vi "phasePlotWrap.vi"(6 "Sampling info":cluster{"Fs":dbl, "#s":dbl}={"Fs"=10000.0, "#s"=1000.0} {"Fs" format="%.2p"}, 8 "Phase Unit":u16(ring) items=["Degree", "Radian"], 9 "Input phase":dbl, 10 "Input frequency":dbl=50.0, 11 "Nominal Frequency":dbl=50.0) -> (3 "Phase waveform":waveform(dbl)(graph))   [LabVIEW 2025]
uses:
  <vilib>/measure/NI_MAPro.lvlib
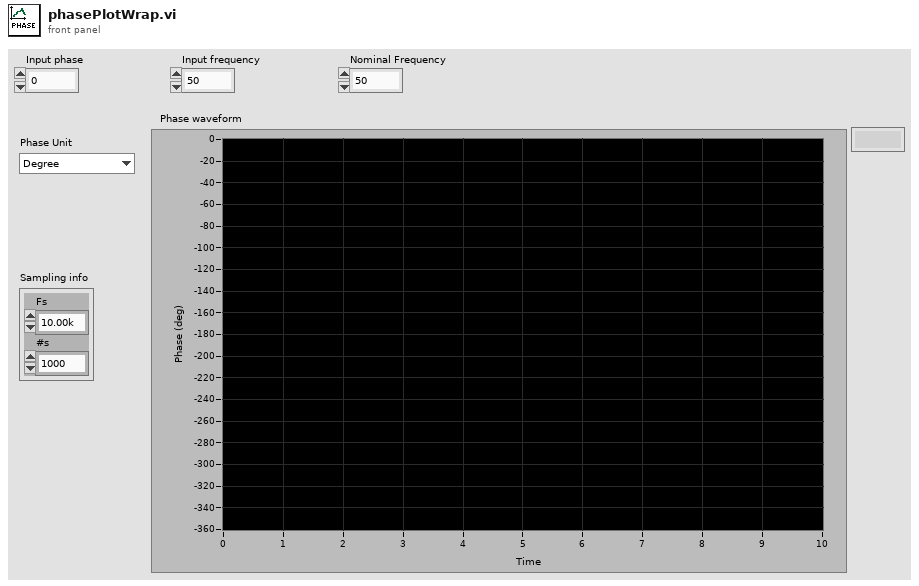
[diagram p1: front panel]
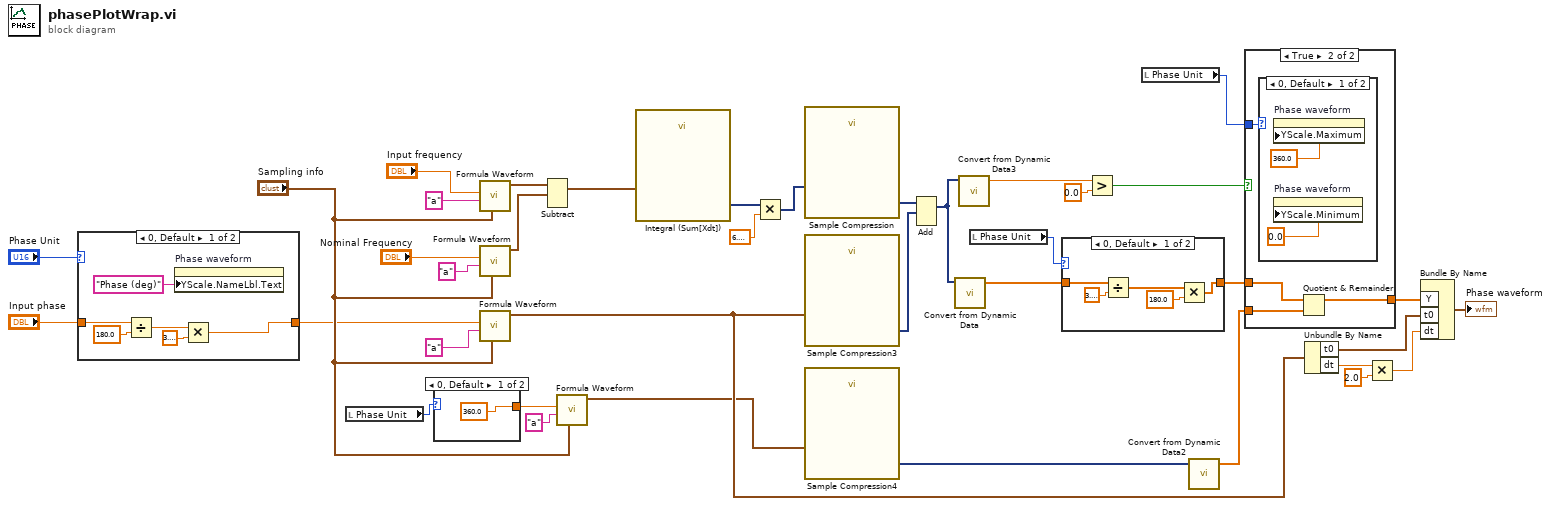
[diagram p0: block diagram]
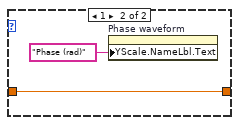
[diagram p2: hidden frame]
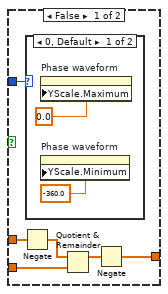
[diagram p3: hidden frame]
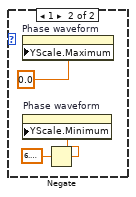
[diagram p4: hidden frame]
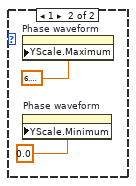
[diagram p5: hidden frame]
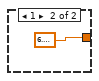
[diagram p6: hidden frame]
diagram:
  n1 = case shown="0, Default" "Phase Unit" {
    tunnel: "Input phase" -> [w42 w45]
    tunnel: [w39 w45] -> w1
    frame 0, Default {
      n2 = Divide(x=w42, y=180.0) -> (x/y=w41:dbl)
      n3 = property on="Phase waveform" class="WFChart (strict)"("YScale.NameLbl.Text"="Phase (deg)" ("Y Scale.Name Label.Text")) -> ()  [unwired: 2 in, 2 out]
      n4 = Multiply(x=w41, y=3.141592653589793) -> (x*y=w39:dbl)
    }
    frame 1 {
      n5 = property on="Phase waveform" class="WFChart (strict)"("YScale.NameLbl.Text"="Phase (rad)" ("Y Scale.Name Label.Text")) -> ()  [unwired: 2 in, 2 out]
    }
  }
  n6 = local read "Phase Unit"() -> (w21:u16)
  n7 = case shown="0, Default" w21 {
    tunnel: [360.0 6.283185307179586] -> w22
    frame 0, Default {
    }
    frame 1 {
    }
  }
  n8 = call <vilib>:"Formula Waveform.vi"("sampling info"="Sampling info", "formula"="a", "amplitude"="Input frequency") -> ("signal out"=w14:waveform(dbl))  [unwired: 7 in, 1 out]
  n9 = call <vilib>:"Formula Waveform.vi"("sampling info"="Sampling info", "formula"="a", "amplitude"="Nominal Frequency") -> ("signal out"=w15:waveform(dbl))  [unwired: 7 in, 1 out]
  n10 = call <vilib>:"Formula Waveform.vi"("sampling info"="Sampling info", "formula"="a", "amplitude"=w1) -> ("signal out"=w31:waveform(dbl))  [unwired: 7 in, 1 out]
  n11 = Subtract(1:w15, 2:w14) -> (0:w16:waveform(dbl))  [unwired: 1 in, 1 out]
  n12 = call <vilib>:"Formula Waveform.vi"("sampling info"="Sampling info", "formula"="a", "amplitude"=w22) -> ("signal out"=w20:waveform(dbl))  [unwired: 7 in, 1 out]
  n13 = call "Integral (Sum[Xdt])"("Signals"=w16) -> ("Result"=w12:dynamicdata)  [unwired: 5 in, 1 out]
  n14 = Multiply(x=w12, y=6.283185307179586) -> (x*y=w10:dynamicdata)
  n15 = call "Sample Compression"("Signals"=w10) -> ("Maximum"=w11:dynamicdata)  [unwired: 8 in, 2 out]
  n16 = call "Sample Compression3"("Signals"=w31) -> ("Maximum"=w27:dynamicdata)  [unwired: 8 in, 2 out]
  n17 = call "Sample Compression4"("Signals"=w20) -> ("Maximum"=w30:dynamicdata)  [unwired: 8 in, 2 out]
  n18 = Add(1:w27, 2:w11) -> (0:w36:dynamicdata)  [unwired: 1 in, 1 out]
  n19 = call "Convert from Dynamic Data"("Dynamic Data Type"=w36) -> ("Array"=w24:dbl[])  [unwired: 3 in]
  n20 = call "Convert from Dynamic Data3"("Dynamic Data Type"=w36) -> ("Scalar"=w37:dbl)  [unwired: 3 in]
  n21 = local read "Phase Unit"() -> (w9:u16)
  n22 = case shown="0, Default" w9 {
    tunnel: w24 -> [w53 w54]
    tunnel: [w50 w54] -> w23
    frame 0, Default {
      n23 = Divide(x=w53, y=3.141592653589793) -> (x/y=w52:dbl[])
      n24 = Multiply(x=w52, y=180.0) -> (x*y=w50:dbl[])
    }
    frame 1 {
    }
  }
  n25 = Greater?(x=w37, y=0.0) -> (0:w26:bool)
  n26 = local read "Phase Unit"() -> (w38:u16)
  n27 = call "Convert from Dynamic Data2"("Dynamic Data Type"=w30) -> ("Array"=w25:dbl[])  [unwired: 3 in]
  n28 = case shown="True" w26 {
    tunnel: w23 -> [w59 w69]
    tunnel: w25 -> [w58 w68]
    tunnel: [w57 w67] -> w28
    tunnel: w38 -> [w55 w66]
    frame False {
      n29 = Negate(x=w59) -> (-x=w60:dbl[])
      n30 = case shown="0, Default" w55 {
        frame 0, Default {
          n31 = property on="Phase waveform" class="WFChart (strict)"("YScale.Maximum"=0.0 ("Y Scale.Range:Maximum")) -> ()  [unwired: 2 in, 2 out]
          n32 = property on="Phase waveform" class="WFChart (strict)"("YScale.Minimum"=-360.0 ("Y Scale.Range:Minimum")) -> ()  [unwired: 2 in, 2 out]
        }
        frame 1 {
          n33 = property on="Phase waveform" class="WFChart (strict)"("YScale.Maximum"=0.0 ("Y Scale.Range:Minimum")) -> ()  [unwired: 2 in, 2 out]
          n34 = Negate(x=6.283185307179586) -> (-x=w63:dbl)
          n35 = property on="Phase waveform" class="WFChart (strict)"("YScale.Minimum"=w63) -> ()  [unwired: 2 in, 2 out]
        }
      }
      n36 = Quotient & Remainder(x=w60, y=w58) -> (x-y*floor(x/y)=w56:dbl[])  [unwired: 1 out]
      n37 = Negate(x=w56) -> (-x=w57:dbl[])
    }
    frame True {
      n38 = case shown="0, Default" w66 {
        frame 0, Default {
          n39 = property on="Phase waveform" class="WFChart (strict)"("YScale.Maximum"=360.0 ("Y Scale.Range:Maximum")) -> ()  [unwired: 2 in, 2 out]
          n40 = property on="Phase waveform" class="WFChart (strict)"("YScale.Minimum"=0.0 ("Y Scale.Range:Minimum")) -> ()  [unwired: 2 in, 2 out]
        }
        frame 1 {
          n41 = property on="Phase waveform" class="WFChart (strict)"("YScale.Maximum"=6.283185307179586) -> ()  [unwired: 2 in, 2 out]
          n42 = property on="Phase waveform" class="WFChart (strict)"("YScale.Minimum"=0.0 ("Y Scale.Range:Minimum")) -> ()  [unwired: 2 in, 2 out]
        }
      }
      n43 = Quotient & Remainder(x=w69, y=w68) -> (x-y*floor(x/y)=w67:dbl[])  [unwired: 1 out]
    }
  }
  n44 = Unbundle By Name(w31) -> ("t0"=w32:timestamp, "dt"=w33:dbl)
  n45 = Multiply(x=w33, y=2.0) -> (x*y=w34:dbl)
  n46 = Bundle By Name("Y"=w28, "t0"=w32, "dt"=w34) -> (→"Phase waveform":waveform(dbl))  [unwired: 1 in]
